vi "CRYCheck Sequance Mismatch.vi"() -> (2 "Match":bool, 3 "Mismatch":bool)   [LabVIEW 2013]
uses:
  CRYProject/CRYProject Editor Global.vi
  CRYMainGlobal.vi
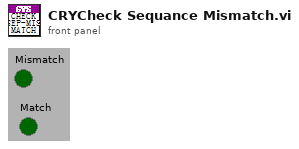
[diagram p1: front panel]
types:
  T1 = typedef "CRYTS.ctl" = cluster{"No.TS":u16, "TS File Path":path, "TS Name":string, "EditStepName":string, "Steps":T2[], "New State":bool, "Change State":bool, "Flattened CurveLib Data":string, "Document Data":string, "EditStepNo":u16, "Operator Start File":string, "Sequence Type":string, "Sequence Language":string}
  T2 = typedef "CRYStep.ctl" = cluster{"No.VI":i32, "Category":string, "StepName":string, "Seq setup flattened":string, "Comment":string, "Steps config.":bool[], "Jump config":i32[], "Start":dbl, "Increment":dbl, "Name":string, "Unit":string, "Y data":u16, "Y prefix":string, "Y dB ref":dbl, "Y unit":string, "Repeat State Array":cluster{"Start":dbl, "Increment":dbl, "Count":i32, "Num":i32}[]}
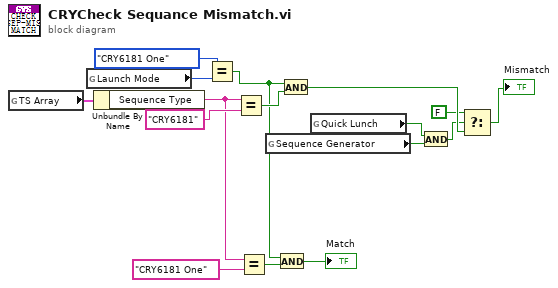
[diagram p0: block diagram]
diagram:
  n1 = global read "CRYProject Editor Global.vi" "TS Array"() -> (w15:T1)
  n2 = global read "CRYMainGlobal.vi" "Launch Mode"() -> (w16:enum32{"CRY6181", "CRY6181 One"})
  n3 = Unbundle By Name(w15) -> ("Sequence Type"=w12:string)
  n4 = Equal?(x=enum32{"CRY6181", "CRY6181 One"}."CRY6181 One", y=w16) -> (x = y?=w8:bool)
  n5 = Equal?(x=w12, y="CRY6181" ("Section")) -> (x = y?=w13:bool)
  n6 = Equal?(x=w12, y="CRY6181 One") -> (x = y?=w10:bool)
  n7 = global read "CRYMainGlobal.vi" "Sequence Generator"() -> (w3:bool)
  n8 = And(x=w8, y=w10) -> (x .and. y?=→"Match":bool)
  n9 = And(x=w8, y=w13) -> (x .and. y?=w7:bool)
  n10 = global read "CRYMainGlobal.vi" "Quick Lunch"() -> (w4:bool)
  n11 = And(x=w4, y=w3) -> (x .and. y?=w2:bool)
  n12 = Select(t=FALSE, s=w2, f=w7) -> (s? t:f=→"Mismatch":bool)
